vi "未命名 4.vi"   [LabVIEW 2018]
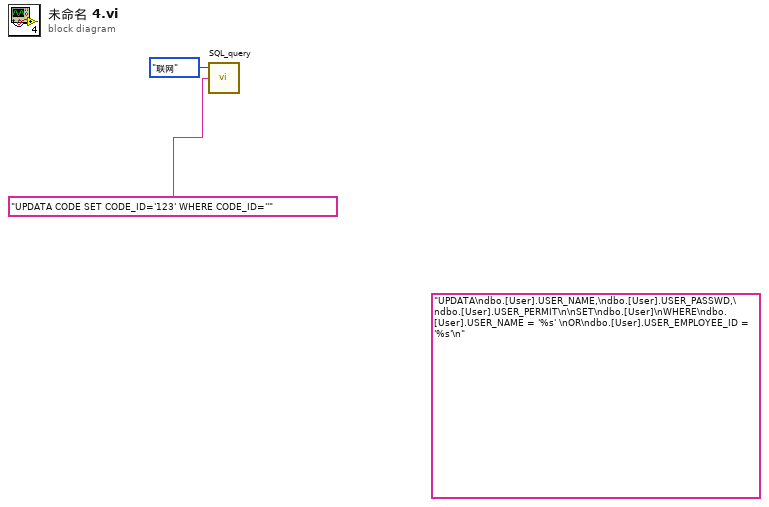
[diagram p0: block diagram]
diagram:
  (unwired) "UPDATA\ndbo.[User].USER_NAME,\ndbo.[User].USER_PASSWD,\ndbo.[User].USER_PERMIT\n\nSET\ndbo.[User]\nWHERE\ndbo.[User].USER_NAME = '%s' \nOR\ndbo.[User].USER_EMPLOYEE_ID = '%s'\n" ("格式字符串")
  n1 = call "SQL_query.vi"("SQL query"="UPDATA CODE SET CODE_ID='123' WHERE CODE_ID=''" ("格式字符串"), "联机模式"=enum16{"单机", "联网"}."联网") -> ()  [unwired: 1 in, 3 out]
